vi "PostAttendanceToDatabase.vi"(8 "error in (no error)":errorcluster) -> (0 "error out":errorcluster)   [LabVIEW 2014, in "FIRST Events API.lvlib"]
uses:
  FIRST Events API.lvlib
  Backend/source/VI Source/FRCts20_Backend_API/FRCts20_Backend_API_Event.ctl
  Backend/source/VI Source/FRCts20_Backend_API/FRCts20_Backend_API_SW.ctl
  Backend/source/VI Source/FRCts20_Backend_API/FRCts20_Backend_API_Command_Event.ctl
  Backend/source/VI Source/FRCts20_Backend_API/FRCts20_Backend_API_Event.vi
  Backend/source/VI Source/FRCts20_Backend_API/FRCts20_Backend_API.lvlib
panel:
  out "Items added to database":i32
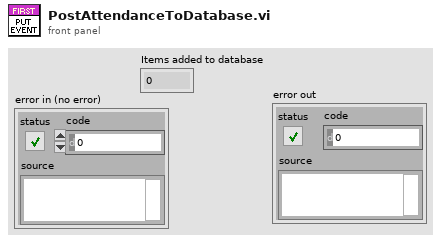
[diagram p1: front panel]
types:
  T1 = typedef "FRCts20_Backend_API.lvlib/FRCts20_Backend_API_EventRoot.ctl" = cluster{"Event":cluster{"Event Index":u32, "EventID":u32, "EventSubtype":string, "EventSubtypeID":u32, "DistrictCode":string, "DistrictID":u32, "Event Name":string, "Venue":string, "City":string, "StateProvince":string, "Country":string, "Start Time":timestamp, "End Time":timestamp, "Year":u32, "NumberOfTeams":u32, "URLTeamlist":string, "EventCode":string, "OpenIssues":u8, "IsLive":bool}[], "APIReturn":string}
  T2 = cluster{"Event Index":u32, "EventID":u32, "EventSubtype":string, "EventSubtypeID":u32, "DistrictCode":string, "DistrictID":u32, "Event Name":string, "Venue":string, "City":string, "StateProvince":string, "Country":string, "Start Time":timestamp, "End Time":timestamp, "Year":u32, "NumberOfTeams":u32, "URLTeamlist":string, "EventCode":string, "OpenIssues":u8, "IsLive":bool}[]
  T3 = typedef "FRCts20_Backend_API.lvlib/FRCts20_Backend_API_SW.ctl" = string
  T4 = cluster{"Team Index":u32, "Team Number":u32, "Team ID":u32, "Team Name":string, "Short Team Name":string, "Nick Name":string, "Robot Name":string, "City":string, "State":string, "Country":string, "Rookie Year":u32, "SWType":T3, "CAN":bool, "Vision":bool, "Kinect":bool, "Tags":string, "Avatar":string, "Events":cluster{"EventIndex":u32, "EventName":string, "IsLive":bool}[]}[]
  T5 = typedef "FRCts20_Backend_API.lvlib/FRCts20_Backend_API_Command_Event.ctl" = string
  T6 = typedef "FRCts20_Backend_API.lvlib/FRCts20_Backend_API_Event.ctl" = cluster{"Event Index":u32, "Name":string, "Start Time":timestamp, "End Time":timestamp, "Teams":cluster{"Team Index":u32, "Team Number":u32, "Requests":cluster{"Request Number":u32, "Description":string}[], "Has Open Issue":bool}[], "SWType":T3, "APIReturn":string}
  T7 = cluster{"Team Index":u32, "Team Number":u32, "Requests":cluster{"Request Number":u32, "Description":string}[], "Has Open Issue":bool}
  T8 = typedef "FRCts20_Backend_API.lvlib/FRCts20_Backend_API_TeamRoot.ctl" = cluster{"Teams":cluster{"Team Index":u32, "Team Number":u32, "Team ID":u32, "Team Name":string, "Short Team Name":string, "Nick Name":string, "Robot Name":string, "City":string, "State":string, "Country":string, "Rookie Year":u32, "SWType":T3, "CAN":bool, "Vision":bool, "Kinect":bool, "Tags":string, "Avatar":string, "Events":cluster{"EventIndex":u32, "EventName":string, "IsLive":bool}[]}[], "APIReturn":string}
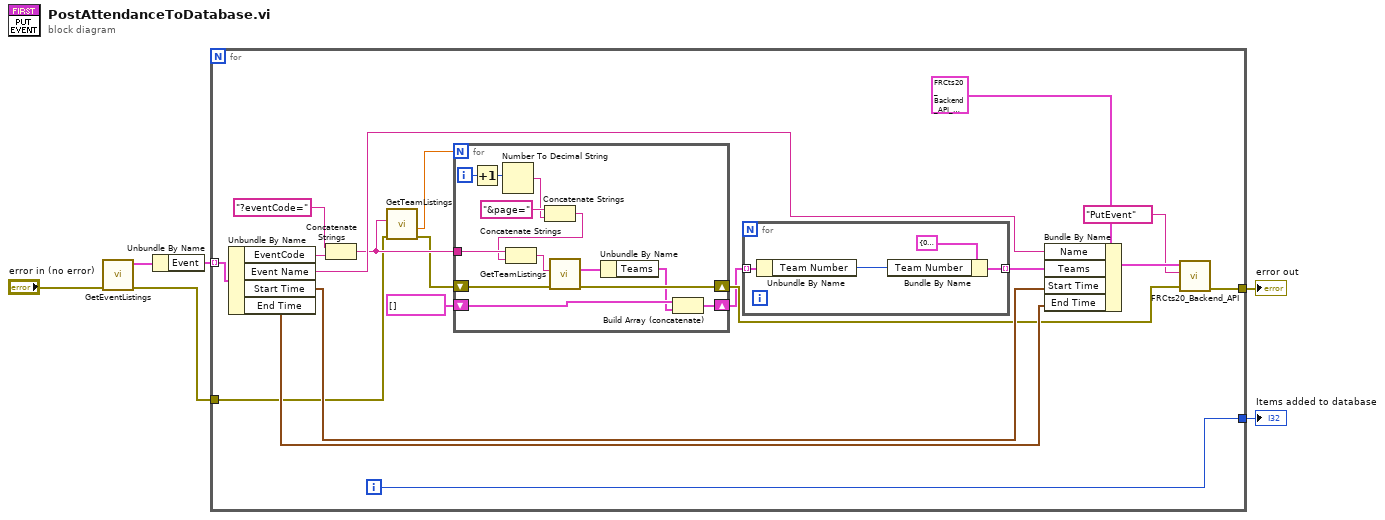
[diagram p0: block diagram]
diagram:
  n1 = call "GetEventListings.vi"("error in (no error)"="error in (no error)") -> ("error out"=w4:errorcluster, "output cluster"=w6:T1)  [unwired: 8 in, 1 out]
  n2 = Unbundle By Name(w6) -> ("Event"=w5:T2)
  n3 = for {
    tunnel: w5 -> [w23] mode=indexing
    tunnel: w4 -> [w16]
    tunnel: [w25] -> w3
    tunnel: [w24] -> w2
    i -> [w24]
    n4 = Unbundle By Name(w23) -> ("EventCode"=w22:string, "Event Name"=w20:string, "Start Time"=w18:timestamp, "End Time"=w19:timestamp)
    n5 = Concatenate Strings("?eventCode=" ("string"), w22) -> (w17:string)
    n6 = call "GetTeamListings.vi"("error in (no error)"=w16, "Append to URL"=w17) -> ("error out"=w15:errorcluster, "pageTotal"=w9:dbl)  [unwired: 7 in, 1 out]
    n7 = for {
      N: w9 -> [_]
      tunnel: w17 -> [w38]
      shift-right: [w35] -> w12
      shift-left: w15 -> [w37]
      shift-right: [w28] -> w8
      shift-left: T4 [] -> [w30]
      i -> [w27]
      n8 = Increment(x=w27) -> (x+1=w26:i32)
      n9 = Number To Decimal String(number=w26) -> (decimal integer string=w33:string)  [unwired: 1 in]
      n10 = Concatenate Strings("&page=" ("string"), w33) -> (w32:string)
      n11 = Concatenate Strings(w38, w32) -> (w31:string)
      n12 = call "GetTeamListings.vi"("error in (no error)"=w37, "Append to URL"=w31) -> ("error out"=w35:errorcluster, "output cluster"=w36:T8)  [unwired: 7 in, 1 out]
      n13 = Unbundle By Name(w36) -> ("Teams"=w29:T4)
      n14 = Build Array (concatenate)(w30, w29) -> (w28:T4)
    }
    n15 = for {
      tunnel: [w40] -> w13 mode=indexing
      tunnel: w8 -> [w39] mode=indexing
      n16 = Unbundle By Name(w39) -> ("Team Number"=w41:u32)
      n17 = Bundle By Name(cluster=T7 {"Team Index"=0, "Team Number"=0, "Requests"=[], "Has Open Issue"=FALSE} ("Team"), "Team Number"=w41) -> (w40:T7)
    }
    n18 = Bundle By Name(cluster=T6 {"Event Index"=0, "Name"="", "Start Time"=timestamp(0 s since 1904-01-01), "End Time"=timestamp(0 s since 1904-01-01), "Teams"=[], "SWType"="", "APIReturn"=""} ("Event In"), "Name"=w20, "Teams"=w13, "Start Time"=w18, "End Time"=w19) -> (w11:T6)
    n19 = call-poly "FRCts20_Backend_API.vi"("error in (no error)"=w12, "Command"=T5 "PutEvent", "Event In"=w11) -> ("error out"=w25:errorcluster)  [unwired: 6 in, 2 out]
  }
  "error out" <- w3
  "Items added to database" <- w2
